vi "Begin.vi"(8 "error in":errorcluster) -> (0 "error out":errorcluster)   [LabVIEW 2018]
doc: "Called before other user functions, this VI is expected to open initial I/O refnums, load in file data, and do all program initialization. Notice that the <B>error out</B> terminal is simply used for data flow. Wiring it to other structures or subVIs ensures that this VI runs first."
uses:
  <vilib>/Rock Robotics/WPI/DriverStation/WPI_DriverStationRobotMode2.ctl
  <vilib>/Rock Robotics/WPI/Joystick/WPI_JoystickDeviceEnum.ctl
  PWF_Venom_LabVIEW/Public/TypeDefs/PwF_Venom_ControlMode.ctl
  PWF_Venom_LabVIEW/Public/TypeDefs/PwF_Venom_BrakeCoastMode.ctl
  <vilib>/Rock Robotics/SystemInterfaces/DIO/FPGA_DIOChannel.ctl
  <vilib>/Rock Robotics/WPI/Encoder/WPI_EncoderType.ctl
  <vilib>/Rock Robotics/WPI/ThirdParty/Phoenix-LabVIEW/Pigeon IMU/CTRE_PigeonIMU_StatusFrameRate.ctl
  <vilib>/Rock Robotics/SystemInterfaces/AI/FPGA_AIChannel.ctl
  <vilib>/Rock Robotics/SystemInterfaces/i2clib/i2c_bus.ctl
  Robot Global Data.vi
  <vilib>/Rock Robotics/WPI/Counter/WPI_CounterDigitalInputToDigitalSource.vi
  <vilib>/Rock Robotics/WPI/ThirdParty/Phoenix-LabVIEW/Pigeon IMU/CTRE_PigeonIMU_Open_CAN.vi
  PWF_Venom_LabVIEW/PwF_Venom.lvlib
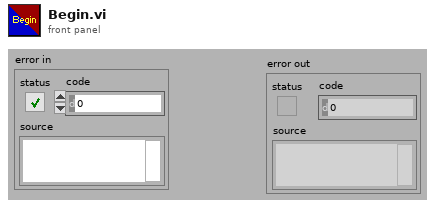
[diagram p1: front panel]
types:
  T1 = typedef "i2c_bus.ctl" = enum16{"I2C On-Board", "I2C MXP", "Invalid"}
  T2 = typedef "FPGA_AIChannel.ctl" = enum8{"AI 0", "AI 1", "AI 2", "AI 3", "AI MXP 0", "AI MXP 1", "AI MXP 2", "AI MXP 3", "Invalid"}
  T3 = typedef "CTRE_PigeonIMU_StatusFrameRate.ctl" = u32
  T4 = typedef "WPI_EncoderType.ctl" = enum16{"1x", "2x", "4x"}
  T5 = typedef "FPGA_DIOChannel.ctl" = enum8{"DIO 0", "DIO 1", "DIO 2", "DIO 3", "DIO 4", "DIO 5", "DIO 6", "DIO 7", "DIO 8", "DIO 9", "DIO MXP 0", "DIO MXP 1", "DIO MXP 2", "DIO MXP 3", "DIO MXP 4", "DIO MXP 5", "DIO MXP 6", "DIO MXP 7", "DIO MXP 8", "DIO MXP 9", "DIO MXP 10", "DIO MXP 11", "DIO MXP 12", "DIO MXP 13", "DIO MXP 14", "DIO MXP 15", "SPI Port CS1", "SPI Port CS2", "SPI Port CS3", "SPI Port MISO", "SPI Port MOSI", "Invalid"}
  T6 = typedef "PwF_Venom.lvlib/PwF_Venom_BrakeCoastMode.ctl" = u8
  T7 = typedef "PwF_Venom.lvlib/PwF_Venom_ControlMode.ctl" = u8
  T8 = typedef "WPI_JoystickDeviceEnum.ctl" = enum16{"USB 0", "USB 1", "USB 2", "USB 3", "USB 4", "USB 5"}
  T9 = typedef "WPI_DriverStationRobotMode2.ctl" = enum16{"Autonomous Disabled", "Autonomous Enabled", "Teleop Disabled", "Teleop Enabled", "Disconnected", "Finish", "Test Disabled", "Test Enabled", "Emergency Stopped"}
  T10 = typedef "WPI_JoystickDevRef.ctl" = cluster{"Device":T8}
  T11 = typedef "CTRE_PigeonIMU_DeviceRef.ctl" = cluster{"DeviceStatus":errorcluster, "Device Number":u8, "Type":T12, "Device ID":u32, "Handle":u64, "UsageFrame":u32, "Library Path":path}
  T12 = typedef "CTRE_PigeonIMU_ConnectionType.ctl" = u32
  T13 = typedef "WPI_DigitalInputDevRef.ctl" = cluster{"DevStatus":errorcluster, "DIO Channel":T5}
  T14 = typedef "WPI_MotorControlDeviceRef.ctl" = cluster{"DeviceStatus":errorcluster, "Type":T15, "PWM":cluster{"PWM Channel":T16, "DeadBand":T17}, "CAN":cluster{"Device Number":u8, "SetOutput VI Ref":variant, "GetOutput VI Ref":variant, "Enable VI Ref":variant, "Disable VI Ref":variant, "Data":variant}, "Invert":bool, "DIO PWM":cluster{"PWM \"Enable\" Channel":T16, "DIOChannel":T5, "PWM Rate":dbl}}
  T15 = typedef "WPI_MotorControlType.ctl" = enum16{"PWM", "CAN", "DIO PWM"}
  T16 = typedef "FPGA_DIOPWMChannel.ctl" = enum8{"PWM 0", "PWM 1", "PWM 2", "PWM 3", "PWM 4", "PWM 5", "PWM 6", "PWM 7", "PWM 8", "PWM 9", "PWM MXP 0", "PWM MXP 1", "PWM MXP 2", "PWM MXP 3", "PWM MXP 4", "PWM MXP 5", "PWM MXP 6", "PWM MXP 7", "PWM MXP 8", "PWM MXP 9", "Invalid"}
  T17 = typedef "WPI_PWMDeadband.ctl" = cluster{"Name":string, "maxPositivePwm":i32, "minPositivePwm":i32, "centerPwm":i32, "maxNegativePwm":i32, "minNegativePwm":i32, "angularRange":u16}
  T18 = typedef "FPGA_CounterEncoderSourceConvertionLVSourceType.ctl" = cluster{"DevStatus":errorcluster, "AnalogTriggerMode?":bool, "DigitalMode":cluster{"DIO Channel":T19}, "AnalogTriggerMode":cluster{"AnalogTriggerIndex":T20, "OutputType":T21}}
  T19 = typedef "FPGA_DIODigitalSourceChannel.ctl" = enum8{"DIO 0", "DIO 1", "DIO 2", "DIO 3", "DIO 4", "DIO 5", "DIO 6", "DIO 7", "DIO 8", "DIO 9", "DIO MXP 0", "DIO MXP 1", "DIO MXP 2", "DIO MXP 3", "DIO MXP 4", "DIO MXP 5", "DIO MXP 6", "DIO MXP 7", "DIO MXP 8", "DIO MXP 9", "DIO MXP 10", "DIO MXP 11", "DIO MXP 12", "DIO MXP 13", "DIO MXP 14", "DIO MXP 15", "SPI Port CS1", "SPI Port CS2", "SPI Port CS3", "SPI Port MISO", "SPI Port MOSI", "Disabled"}
  T20 = typedef "FPGA_AnalogTriggerIndex.ctl" = enum8{"Trig 0", "Trig 1", "Trig 2", "Trig 3", "Trig 4", "Trig 5", "Trig 6", "Trig 7", "Invalid"}
  T21 = typedef "FPGA_AnalogTriggerOutType.ctl" = enum16{"InWindow", "TriggerState", "Rising", "Falling"}
  T22 = typedef "WPI_EncoderDevRef.ctl" = cluster{"DevStatus":errorcluster, "EncoderIndex":T23, "CounterIndex":T24, "DistancePerCount":dbl, "Decoding Type":T4}
  T23 = typedef "FPGA_EncoderIdx.ctl" = enum8{"Enc 0", "Enc 1", "Enc 2", "Enc 3", "Enc 4", "Enc 5", "Enc 6", "Enc 7", "Invalid"}
  T24 = typedef "FPGA_CounterCtrSystemIndex.ctl" = enum8{"Ctr 0", "Ctr 1", "Ctr 2", "Ctr 3", "Ctr 4", "Ctr 5", "Ctr 6", "Ctr 7", "Invalid"}
  T25 = typedef "WPI_AnalogChannelDevRef.ctl" = cluster{"DevStatus":errorcluster, "Analog Channel":T2}
  T26 = typedef "WPI_I2CDevRef.ctl" = cluster{"DevStatus":errorcluster, "Device Address":u8, "Handle":i32, "I2C Bus":T1}
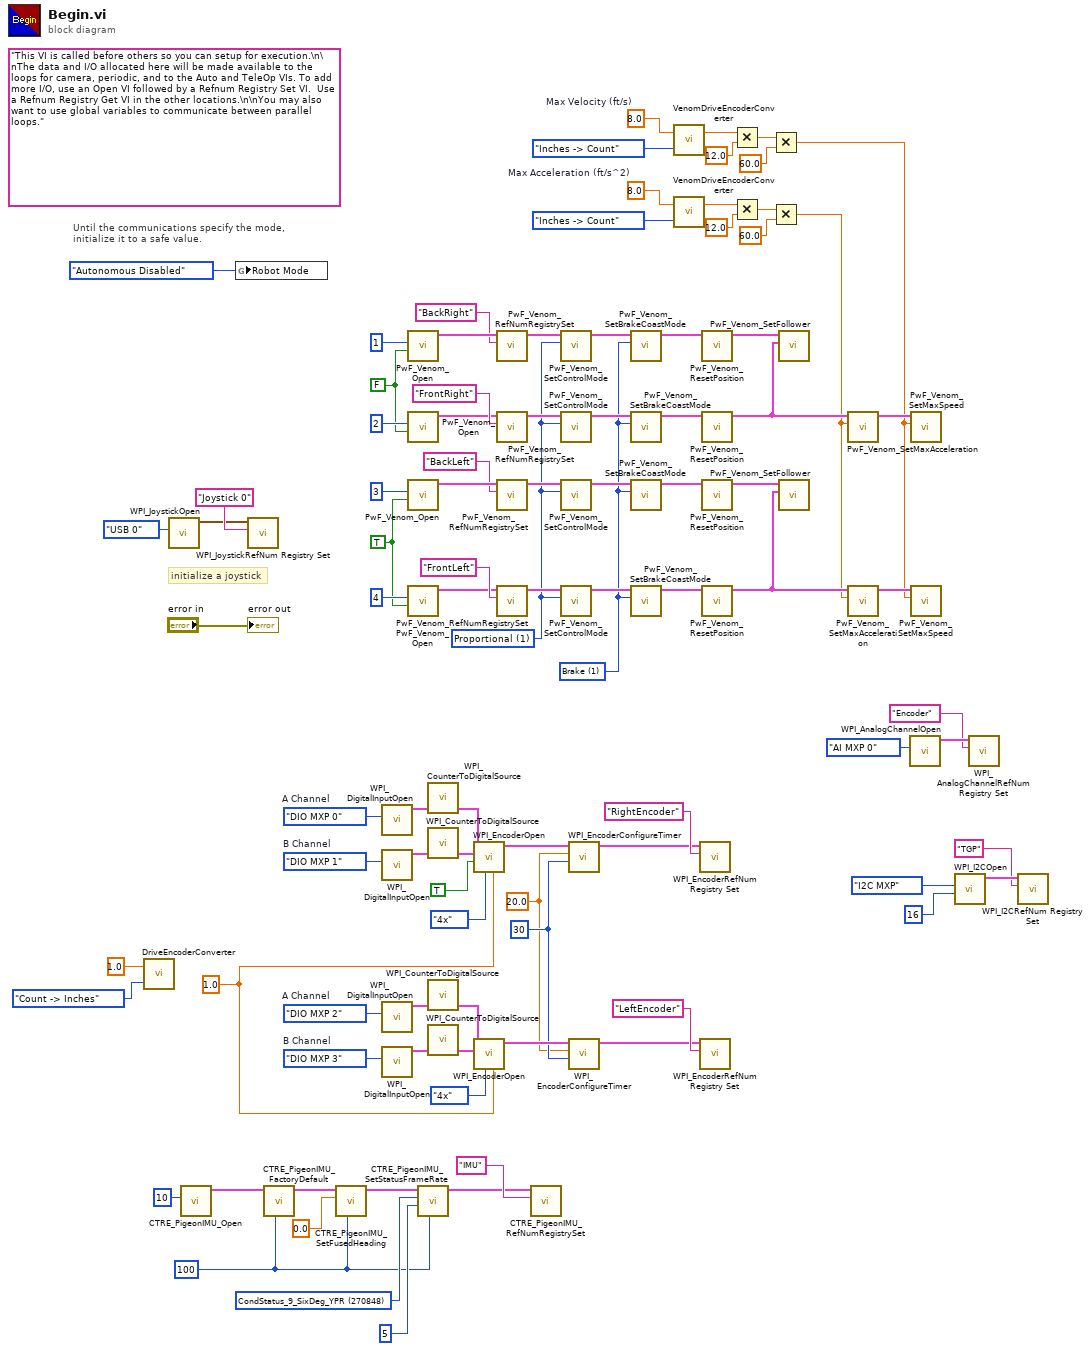
[diagram p0: block diagram]
diagram:
  w17 = 8.0  # Max Acceleration (ft/s^2)
  w18 = 8.0  # Max Velocity (ft/s)
  w34 = T3 270848 items=["CondStatus_1_General"=270336, "CondStatus_9_SixDeg_YPR"=270848, "CondStatus_6_SensorFusion"=270656, "CondStatus_11_GyroAccum"=270976, "CondStatus_2_GeneralCompass"=270400, "CondStatus_3_GeneralAccel"=270464, "CondStatus_10_SixDeg_Quat"=270912, "RawStatus_4_Mag"=265408, "BiasedStatus_2_Gyro"=269376, "BiasedStatus_4_Mag"=269504, "BiasedStatus_6_Accel"=269632] ("StatusFrame")
  w37 = 1.0 ("DistancePerCount")
  w32 = 100 ("timeoutMs")
  w45 = 20.0 ("Minimum Rate")
  w46 = u8 30 ("Number Samples to Average")
  w54 = FPGA_DIOChannel."DIO MXP 3"  # B Channel
  w55 = FPGA_DIOChannel."DIO MXP 2"  # A Channel
  w67 = FPGA_DIOChannel."DIO MXP 1"  # B Channel
  w66 = FPGA_DIOChannel."DIO MXP 0"  # A Channel
  w68 = T6 1 items=["Coast", "Brake"] ("Brake Coast Mode")
  w73 = TRUE ("Invert")
  w74 = FALSE ("Invert")
  w75 = T7 1 items=["Disabled"=0, "Proportional"=1, "Current Control"=3, "Speed Control"=4, "Position Control"=5, "Motion Profile"=6, "Follow The Leader"=7, "Voltage Control"=8] ("Control Mode")
  (unwired) "This VI is called before others so you can setup for execution.\n\nThe data and I/O allocated here will be made available to the loops for camera, periodic, and to the Auto and TeleOp VIs. To add more I/O, use an Open VI followed by a Refnum Registry Set VI.  Use a Refnum Registry Get VI in the other locations.\n\nYou may also want to use global variables to communicate between parallel loops."
  # "initialize a joystick"
  # "Until the communications specify the mode,\ninitialize it to a safe value."
  n1 = call "DriveEncoderConverter.vi"("Mode"=enum16{"Count -> Inches", "Inches -> Count"}."Count -> Inches", "Input"=1.0) -> ()  [unwired: 1 in, 1 out]
  n2 = call <vilib>:"WPI_JoystickOpen.vi"("JoystickDevice"=WPI_JoystickDeviceEnum."USB 0") -> ("JoystickDevRef"=w94:T10)  [unwired: 10 in]
  n3 = call-poly <vilib>:"CTRE_PigeonIMU_Open.vi"("Device Number"=u8 10) -> ("PigeonIMUDevRef"=w41:T11)  [unwired: 9 in, 1 out]
  n4 = global write "Robot Global Data.vi" "Robot Mode"(WPI_DriverStationRobotMode2."Autonomous Disabled" ("Robot Mode")) -> ()
  n5 = call <vilib>:"WPI_JoystickRefNum Registry Set.vi"("refnum name"="Joystick 0", "JoystickDevRef"=w94) -> ()  [unwired: 8 in, 2 out]
  n6 = call <vilib>:"CTRE_PigeonIMU_FactoryDefault.vi"("timeoutMs"=w32, "PigeonIMUDevRef"=w41) -> ("PigeonIMUDevRef"=w39:T11)  [unwired: 8 in, 1 out]
  n7 = call <vilib>:"CTRE_PigeonIMU_SetFusedHeading.vi"("timeoutMs"=w32, "Value"=0.0, "PigeonIMUDevRef 2"=w39) -> ("PigeonIMUDevRef"=w36:T11)  [unwired: 7 in, 1 out]
  n8 = call <vilib>:"WPI_DigitalInputOpen.vi"("DIO Channel"=w66) -> ("DigitalInputDevRef"=w63:T13)  [unwired: 1 in, 9 out]
  n9 = call <vilib>:"WPI_DigitalInputOpen.vi"("DIO Channel"=w67) -> ("DigitalInputDevRef"=w64:T13)  [unwired: 1 in, 9 out]
  n10 = call <vilib>:"WPI_DigitalInputOpen.vi"("DIO Channel"=w55) -> ("DigitalInputDevRef"=w58:T13)  [unwired: 1 in, 9 out]
  n11 = call <vilib>:"WPI_DigitalInputOpen.vi"("DIO Channel"=w54) -> ("DigitalInputDevRef"=w57:T13)  [unwired: 1 in, 9 out]
  n12 = call "PwF_Venom_Open.vi"("Invert"=w74, "Device Number"=u8 1) -> ("Venom Ref"=w91:T14)  [unwired: 8 in, 1 out]
  n13 = call "PwF_Venom_Open.vi"("Invert"=w74, "Device Number"=u8 2) -> ("Venom Ref"=w86:T14)  [unwired: 8 in, 1 out]
  n14 = call "PwF_Venom_Open.vi"("Invert"=w73, "Device Number"=u8 3) -> ("Venom Ref"=w85:T14)  [unwired: 8 in, 1 out]
  n15 = call "PwF_Venom_Open.vi"("Invert"=w73, "Device Number"=u8 4) -> ("Venom Ref"=w80:T14)  [unwired: 8 in, 1 out]
  n16 = call <vilib>:"CTRE_PigeonIMU_SetStatusFrameRate.vi"("timeoutMs"=w32, "Period (ms)"=i16 5, "StatusFrame"=w34, "PigeonIMUDevRef"=w36) -> ("PigeonIMUDevRef"=w35:T11)  [unwired: 6 in, 1 out]
  n17 = call-poly <vilib>:"WPI_CounterToDigitalSource.vi"("DigitalInputDevRef"=w63) -> ("Digital Source"=w62:T18)  [unwired: 6 out]
  n18 = call-poly <vilib>:"WPI_CounterToDigitalSource.vi"("DigitalInputDevRef"=w64) -> ("Digital Source"=w65:T18)  [unwired: 6 out]
  n19 = call-poly <vilib>:"WPI_CounterToDigitalSource.vi"("DigitalInputDevRef"=w58) -> ("Digital Source"=w59:T18)  [unwired: 6 out]
  n20 = call-poly <vilib>:"WPI_CounterToDigitalSource.vi"("DigitalInputDevRef"=w57) -> ("Digital Source"=w56:T18)  [unwired: 6 out]
  n21 = call <vilib>:"WPI_EncoderOpen.vi"("DistancePerCount"=w37, "Decoding Type"=WPI_EncoderType."4x", "Invert Direction (False)"=TRUE, "BSource"=w65, "ASource"=w62) -> ("EncoderDevRef"=w49:T22)  [unwired: 3 in, 3 out]
  n22 = call <vilib>:"WPI_EncoderOpen.vi"("DistancePerCount"=w37, "Decoding Type"=WPI_EncoderType."4x", "BSource"=w56, "ASource"=w59) -> ("EncoderDevRef"=w48:T22)  [unwired: 4 in, 3 out]
  n23 = call "PwF_Venom_RefNumRegistrySet.vi"("refnum name"="BackRight", "PwFVenomDevRefIn"=w91) -> ("PwFVenomDevRefOut"=w77:T14)  [unwired: 8 in, 1 out]
  n24 = call "PwF_Venom_RefNumRegistrySet.vi"("refnum name"="FrontRight", "PwFVenomDevRefIn"=w86) -> ("PwFVenomDevRefOut"=w78:T14)  [unwired: 8 in, 1 out]
  n25 = call "PwF_Venom_RefNumRegistrySet.vi"("refnum name"="BackLeft", "PwFVenomDevRefIn"=w85) -> ("PwFVenomDevRefOut"=w76:T14)  [unwired: 8 in, 1 out]
  n26 = call "PwF_Venom_RefNumRegistrySet.vi"("refnum name"="FrontLeft", "PwFVenomDevRefIn"=w80) -> ("PwFVenomDevRefOut"=w79:T14)  [unwired: 8 in, 1 out]
  n27 = call <vilib>:"CTRE_PigeonIMU_RefNumRegistrySet.vi"("refnum name"="IMU", "PigeonIMUDevRef"=w35) -> ()  [unwired: 8 in, 2 out]
  n28 = call "PwF_Venom_SetControlMode.vi"("Control Mode"=w75, "PwFVenomDevRefIn"=w77) -> ("PwFVenomDevRefOut"=w72:T14)  [unwired: 8 in, 1 out]
  n29 = call "PwF_Venom_SetControlMode.vi"("Control Mode"=w75, "PwFVenomDevRefIn"=w78) -> ("PwFVenomDevRefOut"=w71:T14)  [unwired: 8 in, 1 out]
  n30 = call "PwF_Venom_SetControlMode.vi"("Control Mode"=w75, "PwFVenomDevRefIn"=w76) -> ("PwFVenomDevRefOut"=w70:T14)  [unwired: 8 in, 1 out]
  n31 = call "PwF_Venom_SetControlMode.vi"("Control Mode"=w75, "PwFVenomDevRefIn"=w79) -> ("PwFVenomDevRefOut"=w69:T14)  [unwired: 8 in, 1 out]
  n32 = call <vilib>:"WPI_EncoderConfigureTimer.vi"("Number Samples to Average"=w46, "Minimum Rate"=w45, "EncoderDevRef"=w49) -> ("EncoderDevRef"=w50:T22)  [unwired: 7 in, 1 out]
  n33 = call <vilib>:"WPI_EncoderConfigureTimer.vi"("Number Samples to Average"=w46, "Minimum Rate"=w45, "EncoderDevRef"=w48) -> ("EncoderDevRef"=w47:T22)  [unwired: 7 in, 1 out]
  n34 = call "PwF_Venom_SetBrakeCoastMode.vi"("Brake Coast Mode"=w68, "PwFVenomDevRefIn"=w72) -> ("PwFVenomDevRefOut"=w30:T14)  [unwired: 8 in, 1 out]
  n35 = call "PwF_Venom_SetBrakeCoastMode.vi"("Brake Coast Mode"=w68, "PwFVenomDevRefIn"=w71) -> ("PwFVenomDevRefOut"=w31:T14)  [unwired: 8 in, 1 out]
  n36 = call "PwF_Venom_SetBrakeCoastMode.vi"("Brake Coast Mode"=w68, "PwFVenomDevRefIn"=w70) -> ("PwFVenomDevRefOut"=w29:T14)  [unwired: 8 in, 1 out]
  n37 = call "PwF_Venom_SetBrakeCoastMode.vi"("Brake Coast Mode"=w68, "PwFVenomDevRefIn"=w69) -> ("PwFVenomDevRefOut"=w28:T14)  [unwired: 8 in, 1 out]
  n38 = call "VenomDriveEncoderConverter.vi"("Mode"=enum16{"Count -> Inches", "Inches -> Count"}."Inches -> Count", "Input"=w18) -> ("Output"=w19:dbl)  [unwired: 1 in]
  n39 = call "VenomDriveEncoderConverter.vi"("Mode"=enum16{"Count -> Inches", "Inches -> Count"}."Inches -> Count", "Input"=w17) -> ("Output"=w16:dbl)  [unwired: 1 in]
  n40 = call <vilib>:"WPI_EncoderRefNum Registry Set.vi"("refnum name"="RightEncoder", "EncoderDevRef"=w50) -> ()  [unwired: 8 in, 2 out]
  n41 = call <vilib>:"WPI_EncoderRefNum Registry Set.vi"("refnum name"="LeftEncoder", "EncoderDevRef"=w47) -> ()  [unwired: 8 in, 2 out]
  n42 = call "PwF_Venom_ResetPosition.vi"("PwFVenomDevRefIn"=w30) -> ("PwFVenomDevRefOut"=w27:T14)  [unwired: 9 in, 1 out]
  n43 = call "PwF_Venom_ResetPosition.vi"("PwFVenomDevRefIn"=w31) -> ("PwFVenomDevRefOut"=w25:T14)  [unwired: 9 in, 1 out]
  n44 = call "PwF_Venom_ResetPosition.vi"("PwFVenomDevRefIn"=w29) -> ("PwFVenomDevRefOut"=w26:T14)  [unwired: 9 in, 1 out]
  n45 = call "PwF_Venom_ResetPosition.vi"("PwFVenomDevRefIn"=w28) -> ("PwFVenomDevRefOut"=w11:T14)  [unwired: 9 in, 1 out]
  n46 = Multiply(x=w19, y=12.0) -> (x*y=w22:dbl)
  n47 = Multiply(x=w16, y=12.0) -> (x*y=w13:dbl)
  n48 = Multiply(x=w22, y=60.0) -> (x*y=w8:dbl)
  n49 = Multiply(x=w13, y=60.0) -> (x*y=w9:dbl)
  n50 = call "PwF_Venom_SetFollower.vi"("LeaderDevRef"=w25, "PwFVenomDevRefIn"=w27) -> ()  [unwired: 8 in, 2 out]
  n51 = call "PwF_Venom_SetFollower.vi"("LeaderDevRef"=w11, "PwFVenomDevRefIn"=w26) -> ()  [unwired: 8 in, 2 out]
  n52 = call "PwF_Venom_SetMaxAcceleration.vi"("Limit"=w9, "PwFVenomDevRefIn"=w25) -> ("PwFVenomDevRefOut"=w24:T14)  [unwired: 8 in, 1 out]
  n53 = call "PwF_Venom_SetMaxAcceleration.vi"("Limit"=w9, "PwFVenomDevRefIn"=w11) -> ("PwFVenomDevRefOut"=w10:T14)  [unwired: 8 in, 1 out]
  n54 = call <vilib>:"WPI_AnalogChannelOpen.vi"("Analog Channel"=FPGA_AIChannel."AI MXP 0") -> ("AIDeviceRef"=w6:T25)  [unwired: 9 in, 1 out]
  n55 = call "PwF_Venom_SetMaxSpeed.vi"("Limit"=w8, "PwFVenomDevRefIn"=w24) -> ()  [unwired: 8 in, 2 out]
  n56 = call "PwF_Venom_SetMaxSpeed.vi"("Limit"=w8, "PwFVenomDevRefIn"=w10) -> ()  [unwired: 8 in, 2 out]
  n57 = call <vilib>:"WPI_I2COpen.vi"("Device Address"=u8 16, "I2C Bus"=i2c_bus."I2C MXP") -> ("I2CDevRef"=w2:T26)  [unwired: 8 in, 1 out]
  n58 = call <vilib>:"WPI_AnalogChannelRefNum Registry Set.vi"("refnum name"="Encoder", "AIDeviceRef"=w6) -> ()  [unwired: 8 in, 2 out]
  n59 = call <vilib>:"WPI_I2CRefNum Registry Set.vi"("refnum name"="TGP", "I2CDevRef"=w2) -> ()  [unwired: 8 in, 2 out]
  "error out" <- "error in"
